vi "P1E2 ZAL 2015640414.vi"() -> ()   [LabVIEW 2016]
panel:
  out "DISPLAY 3":T1
  out "DISPLAY 2":T1
  out "DISPLAY":T1
  in  "B6":bool
  in  "B5":bool
  in  "B4":bool
  in  "B3":bool
  in  "B2":bool
  in  "B1":bool
  in  "B0":bool
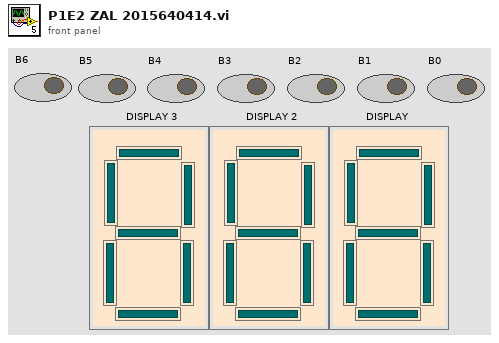
[diagram p1: front panel]
types:
  T1 = cluster{"SA":bool, "SB":bool, "SC":bool, "SD":bool, "SE":bool, "SF":bool, "SG":bool}
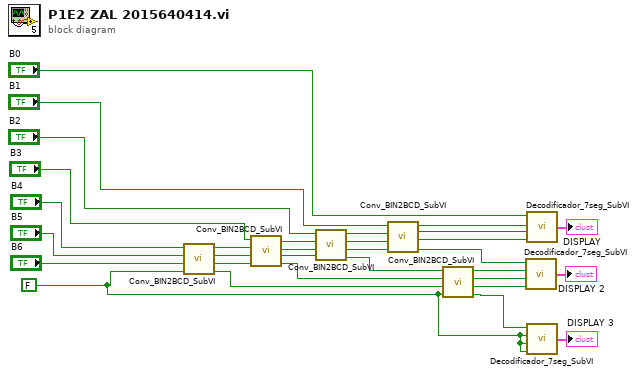
[diagram p0: block diagram]
diagram:
  w4 = FALSE ("W")
  n1 = call "Conv_BIN2BCD_SubVI.vi"("W"=w4, "X"="B6", "Y"="B5", "Z"="B4") -> ("A"=w10:bool, "B"=w28:bool, "C"=w27:bool, "D"=w26:bool)
  n2 = call "Conv_BIN2BCD_SubVI.vi"("W"=w28, "X"=w27, "Y"=w26, "Z"="B3") -> ("A"=w11:bool, "B"=w24:bool, "C"=w23:bool, "D"=w22:bool)
  n3 = call "Conv_BIN2BCD_SubVI.vi"("W"=w24, "X"=w23, "Y"=w22, "Z"="B2") -> ("A"=w12:bool, "B"=w20:bool, "C"=w19:bool, "D"=w18:bool)
  n4 = call "Conv_BIN2BCD_SubVI.vi"("W"=w20, "X"=w19, "Y"=w18, "Z"="B1") -> ("A"=w6:bool, "B"=w16:bool, "C"=w15:bool, "D"=w14:bool)
  n5 = call "Conv_BIN2BCD_SubVI.vi"("W"=w4, "X"=w10, "Y"=w11, "Z"=w12) -> ("A"=w5:bool, "B"=w9:bool, "C"=w8:bool, "D"=w7:bool)
  n6 = call "Decodificador_7seg_SubVI.vi"("A"=w9, "B"=w8, "C"=w7, "D"=w6) -> ("DISPLAY"=→"DISPLAY 2":T1)
  n7 = call "Decodificador_7seg_SubVI.vi"("A"=w16, "B"=w15, "C"=w14, "D"="B0") -> ("DISPLAY"=→"DISPLAY":T1)
  n8 = call "Decodificador_7seg_SubVI.vi"("A"=w4, "B"=w4, "C"=w4, "D"=w5) -> ("DISPLAY"=→"DISPLAY 3":T1)
